vi "Load_Map.vi"(7 "error in (no error)":errorcluster) -> (0 "error out":errorcluster, 2 "image size":i32[](array[numeric]), 3 "Image Out":T1(plugin-control))   [LabVIEW 2020]
doc: "Allows the user to select an image file as a map of the library.\nOutputs the resolution of the map."
panel:
  out "Y Resolution":i32
  out "X Resolution":i32
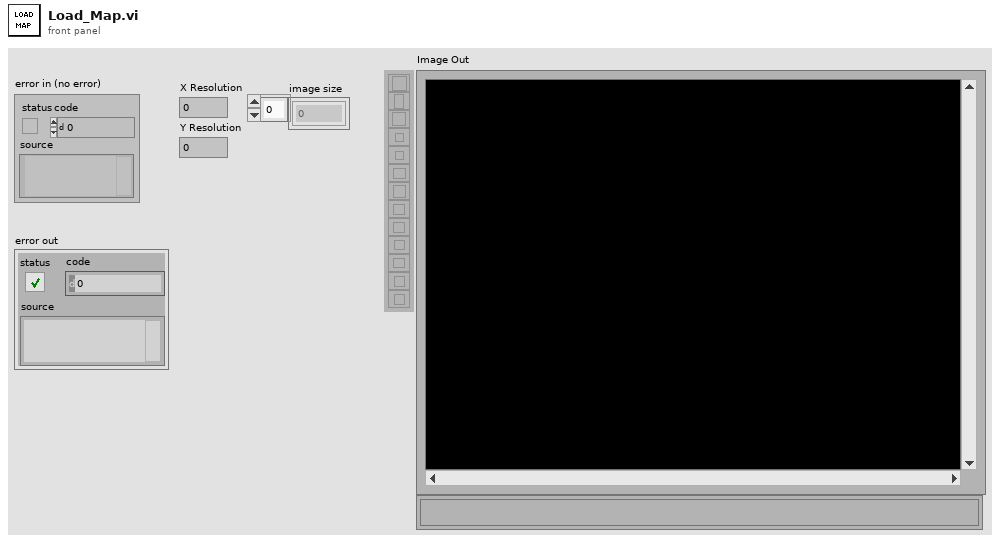
[diagram p1: front panel]
types:
  T1 = typedef "IMAQ Image.ctl" = refnum<image>
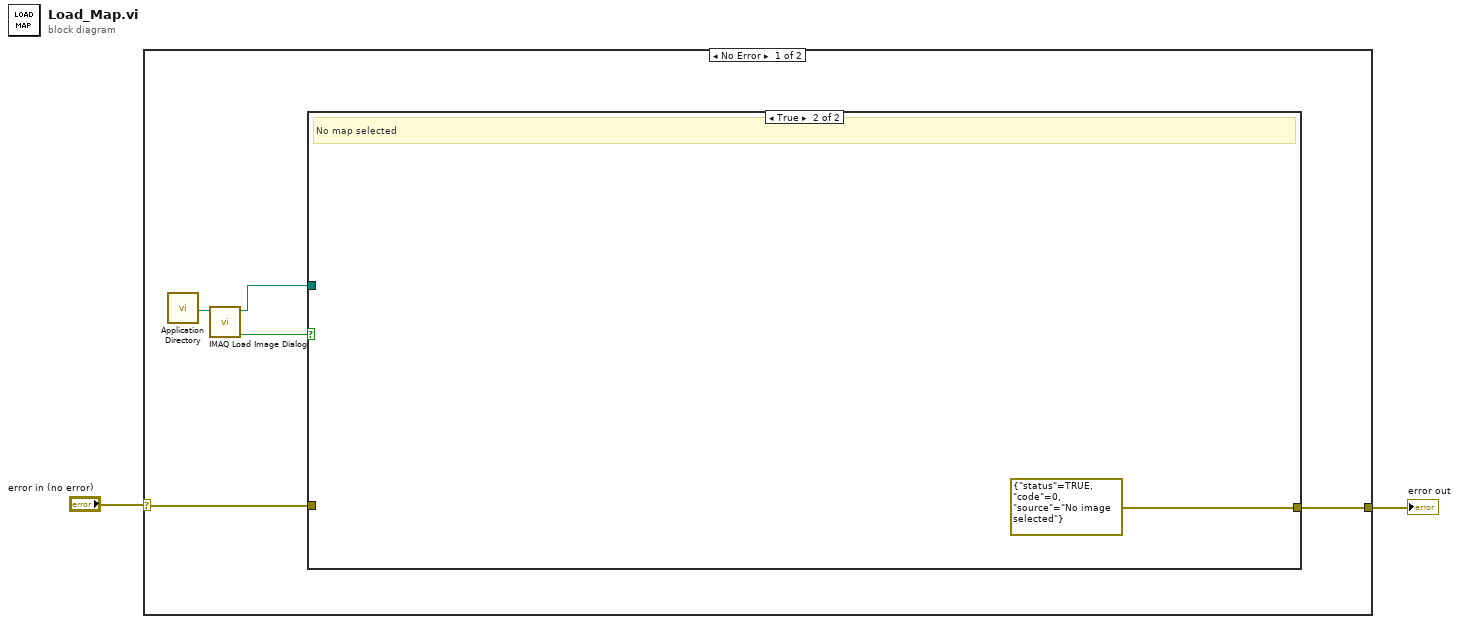
[diagram p0: block diagram]
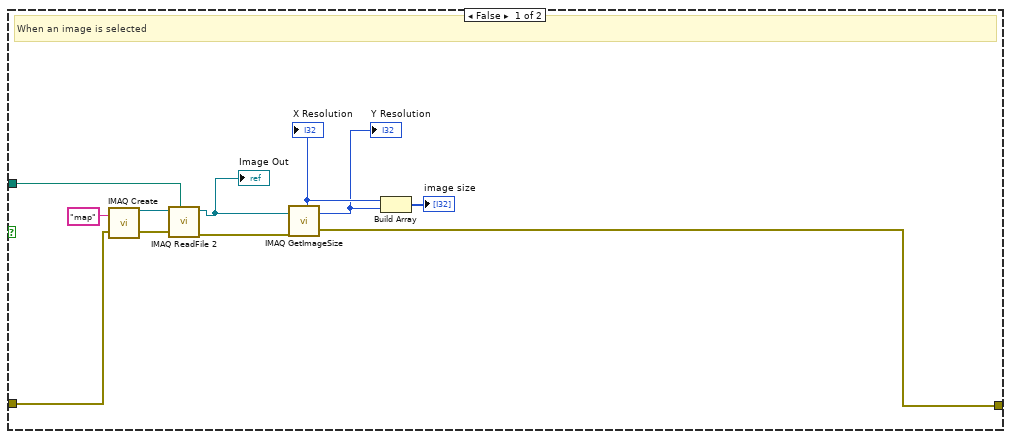
[diagram p2: hidden frame]
diagram:
  n1 = case shown="No Error" "error in (no error)" {
    selector: "error in (no error)" -> [w4 w20]
    tunnel: [w3 w20] -> w1
    frame No Error {
      n2 = call <vilib>:"Application Directory.vi"() -> ("Application Directory"=w7:path)
      n3 = call "IMAQ Load Image Dialog"("Start Path"=w7) -> ("Cancelled?"=w6:bool, "Path"=w5:path)  [unwired: 8 in, 1 out]
      n4 = case shown="True" w6 {
        tunnel: w5 -> [w16 _]
        tunnel: w4 -> [w14 _]
        tunnel: [w13 errorcluster {"status"=TRUE, "code"=0, "source"="No image selected"} ("error out")] -> w3
        frame False {
          # "When an image is selected"
          n5 = call "IMAQ Create"("Image Name"="map", "error in (no error)"=w14) -> ("New Image"=w18:T1, "error out"=w15:errorcluster)  [unwired: 3 in]
          n6 = call "IMAQ ReadFile 2"("File Path"=w16, "error in (no error)"=w15, "Image"=w18) -> ("error out"=w9:errorcluster, "Image Out"=w8:T1)  [unwired: 4 in, 3 out]
          "Image Out" <- w8
          n7 = call "IMAQ GetImageSize"("Image"=w8, "error in (no error)"=w9) -> ("Y Resolution"=w11:i32, "X Resolution"=w12:i32, "error out"=w13:errorcluster)  [unwired: 2 in]
          "X Resolution" <- w12
          "Y Resolution" <- w11
          n8 = Build Array(w12, w11) -> (→"image size":i32[])
        }
        frame True {
          # "No map selected"
        }
      }
    }
    frame Error {
    }
  }
  "error out" <- w1
